vi "BenchConfig_Save.vi"(8 "error in (no error)":errorcluster, 11 "BenchConfig":T1) -> (0 "error out":errorcluster)   [LabVIEW 2013]
uses:
  BenchConfig.ctl
panel:
  # "A configurer"
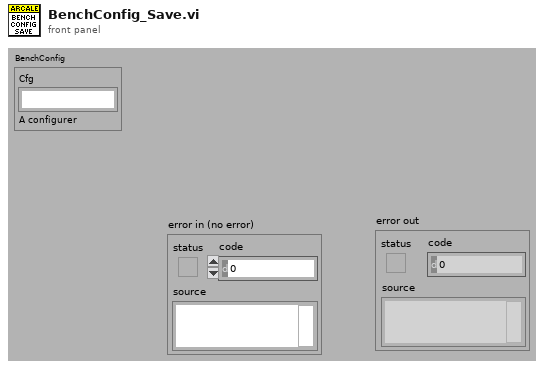
[diagram p1: front panel]
types:
  T1 = typedef "BenchConfig.ctl" = cluster{"Cfg":string}
  T2 = enum16{"open", "replace", "create", "open or create", "replace or create", "replace or create with confirmation"}
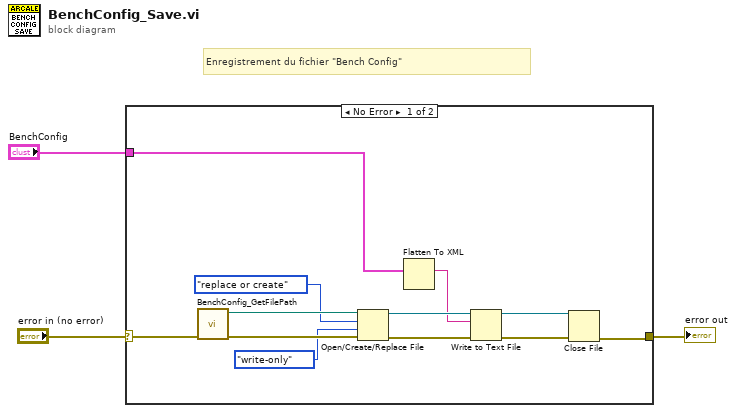
[diagram p0: block diagram]
diagram:
  # "Enregistrement du fichier \"Bench Config\""
  n1 = case shown="No Error" "error in (no error)" {
    selector: "error in (no error)" -> [w15 w16]
    tunnel: [w4 w16] -> w2
    tunnel: "BenchConfig" -> [w8 _]
    frame No Error {
      n2 = call "BenchConfig_GetFilePath.vi"("error in (no error)"=w15) -> ("error out"=w14:errorcluster, "BenchConfigFilePath"=w13:path)  [unwired: 9 in]
      n3 = Open/Create/Replace File(file path (use dialog)=w13, error in=w14, operation (0:open)=T2."replace or create", access (0:read/write)=enum16{"read/write", "read-only", "write-only"}."write-only") -> (refnum out=w9:refnum<file>, error out=w10:errorcluster)  [unwired: 2 in, 1 out]
      n4 = Flatten To XML(anything=w8) -> (xml string=w7:string)
      n5 = Write to Text File(file (use dialog)=w9, text=w7, error in=w10) -> (refnum out=w5:refnum<file>, error out=w6:errorcluster)  [unwired: 1 in, 1 out]
      n6 = Close File(refnum=w5, error in=w6) -> (error out=w4:errorcluster)  [unwired: 1 out]
    }
    frame Error {
    }
  }
  "error out" <- w2
